vi "Vision Processing.vi"(8 "error in (no error)":errorcluster, 11 "Image Size":T1=enum."320x240") -> ()   [LabVIEW 2017]
uses:
  Vision Support Code/Camera Types.ctl
  <vilib>/Rock Robotics/WPI/Camera/WPI_CameraImageSize.ctl
  <vilib>/Rock Robotics/WPI/Camera/WPI_CameraWhite Balance Values.ctl
  <vilib>/Rock Robotics/WPI/Camera/WPI_CameraExposure Values.ctl
  <vilib>/Rock Robotics/WPI/Camera/WPI_CameraFrameRate.ctl
  Robot Global Data.vi
  <vilib>/Rock Robotics/Network Tables/NT Write Number.vi
  <vilib>/vision/NI_Vision_Development_Module.lvlib
panel:
  in  "Image Size 2":T1=enum."320x240"
  in  "Min Component %":dbl=15.0
  out "loop ms":u32
  in  "Display Original":bool
  in  "Display Mask":bool
  out "Instructions:":string="Connect a USB or IP camera to your roboRIO. If using a ring light and retroreflective tape, use Camera Settings outside the loop create a dark image with bright and colorful stripes. If used wihtout a ring light, brighten the images so that stripes are visible.\n\nLED Color can encoded as HSL or related color modes. Calibrate to the same color as the strips being reflected to the camera. Unlike the desktop example, this LED color must be set by hand. You can also put the calibration on the dashboard and send the LED Color to the RT code using Network Tables.\n\nThe Display buttons affects whether images are displayed on the panel. It takes quite a bit of CPU  to compress and transmit the images for display.\n\nAdjust Score Cutoff to make the code more or less picky. If the color is not very unique, you may need to increase the number of particles considered. The diagram uses a Size Limit to ignore colored things that are too small. You may need to adjust it if you are targetting from far away.\n\nResults give you the distance to the target, the center and box in a normalized (-1 to 1) and pixel coordinates.\n\nBe sure to read about setting camera exposure and brightness to help simplify your image and acquire color saturated images.\n\nThere are lots of comments on the diagram to explain the code."
  in  "Color Mode":u16(ring)=2 items=["RGB", "HSL", "HSV", "HSI"]
  in  "Particles":dbl=5.0
  in  "Score Cutoff %":dbl=75.0
  in  "Camera Type":T2=enum."MS HD3000 square"
  out "Result":T3 {"Score" format="%#_3g"; "Pixels"."Rectangle"."Numeric 5" format="%#_3g"; "Pixels"."Rectangle"."Numeric 3" format="%#_3g"; "Pixels"."Rectangle"."Numeric 2" format="%#_3g"; "Pixels"."Rectangle"."Numeric" format="%#_3g"; "Normalized"."Rectangle"."Numeric 5" format="%#_2g"; "Normalized"."Rectangle"."Numeric 3" format="%#_2g"; "Normalized"."Rectangle"."Numeric 2" format="%#_2g"; "Normalized"."Rectangle"."Numeric" format="%#_2g"; "Normalized"."Center"."?" format="%#_3g"; "Normalized"."Center"."?" format="%#_3g"; "Distance (ft)" format="%#_3g"}
  out "Qualified Particles":i32
  in  "LED Color":T4={"Hue"={107.81818389892578, 139.81818389892578}, "Sat"={176.07142857142858, 255.0}, "Val"={40.53571428571429, 255.0}} {"Hue" scale=0.0..255.0 scale format="%#_3g"}
  out "Mask":T5(plugin-control)
  out "Original Image":T5(plugin-control)
  # "Good target, distance ft"
  # "Bad target"
  # "Score in %"
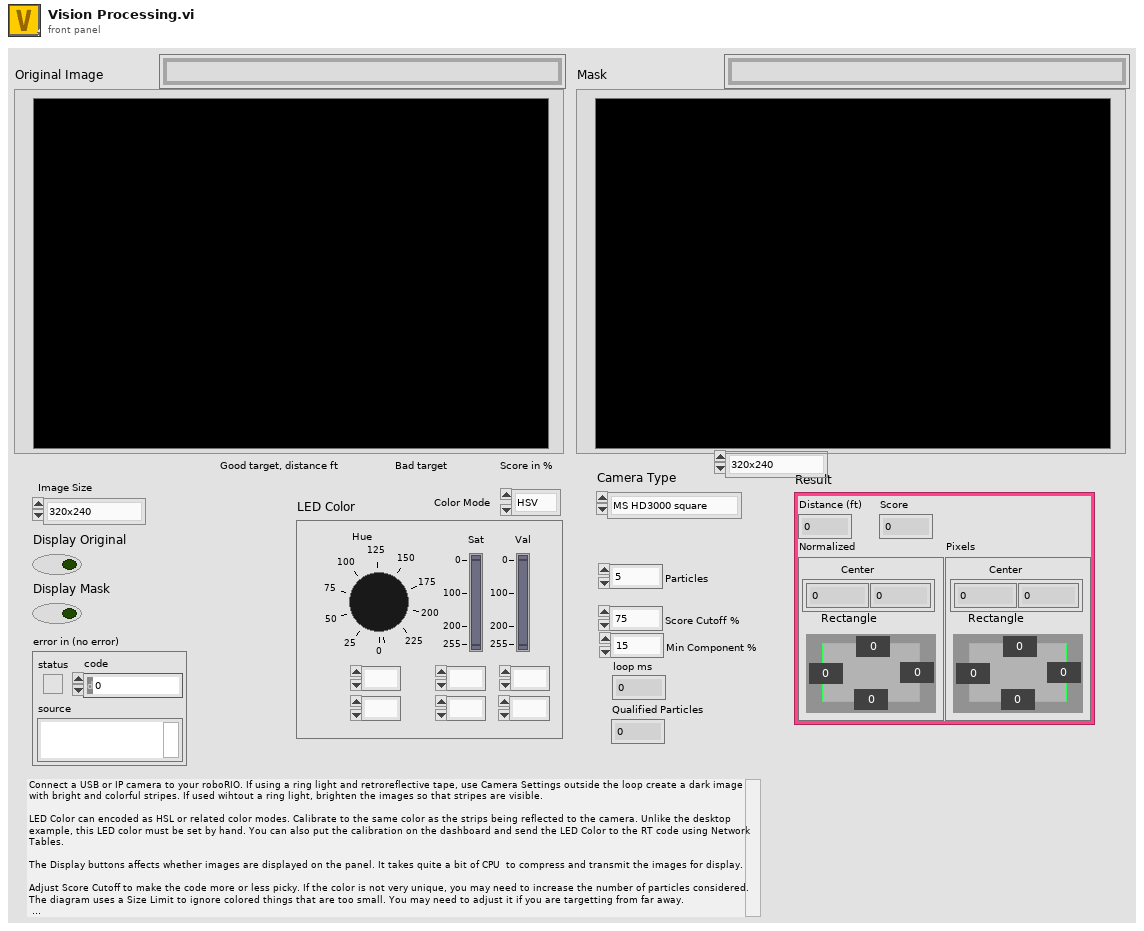
[diagram p1: front panel]
types:
  T1 = typedef "WPI_CameraImageSize.ctl" = enum16{"640x480", "320x240", "160x120", "Custom"}
  T2 = typedef "Camera Types.ctl" = enum16{"206", "1011", "1013", "MS HD3000 square", "MS HD3000 640x480"}
  T3 = cluster{"Distance (ft)":dbl, "Score":dbl, "Normalized":cluster{"Center":cluster{dbl, dbl}, "Rectangle":cluster{"Numeric":dbl, "Numeric 2":dbl, "Numeric 3":dbl, "Numeric 5":dbl}}, "Pixels":cluster{"Center":cluster{dbl, dbl}, "Rectangle":cluster{"Numeric":dbl, "Numeric 2":dbl, "Numeric 3":dbl, "Numeric 5":dbl}}}
  T4 = cluster{"Hue":cluster{dbl, dbl}, "Sat":cluster{dbl, dbl}, "Val":cluster{dbl, dbl}}
  T5 = typedef "IMAQ Image.ctl" = refnum<image>
  T6 = typedef "WPI_CameraFrameRate.ctl" = u32
  T7 = typedef "WPI_CameraExposure Values.ctl" = enum16{"Auto", "Flicker-free 50 Hz", "Flicker-free 60 Hz", "Hold current", "Custom"}
  T8 = typedef "WPI_CameraWhite Balance Values.ctl" = enum16{"Auto", "Fixed indoor", "Fixed outdoor 1", "Fixed outdoor 2", "Fixed fluorescent 1", "Fixed fluorescent 2", "Hold current", "Custom"}
  T9 = typedef "Particle Parameters" = i32
  T10 = typedef "Image Type" = u32
  T11 = typedef "WPI_CameraDevRef.ctl" = cluster{"Camera Address":string, "CameraStatus":errorcluster}
  T12 = cluster{"Score":dbl, "Rect":cluster{"Left":dbl, "Top":dbl, "Right":dbl, "Bottom":dbl}, "Full Scores":cluster{"Aspect Ratio":dbl, "Top Position":dbl, "Bottom Position":dbl, "Left Gap":dbl, "Width":dbl, "Height Ratio":dbl}}[]
  T13 = cluster{"Score":dbl, "Rect":cluster{"Left":dbl, "Top":dbl, "Right":dbl, "Bottom":dbl}, "Full Scores":cluster{"Aspect Ratio":dbl, "Top Position":dbl, "Bottom Position":dbl, "Left Gap":dbl, "Width":dbl, "Height Ratio":dbl}}
  T14 = cluster{"Left":dbl, "Top":dbl, "Right":dbl, "Bottom":dbl}
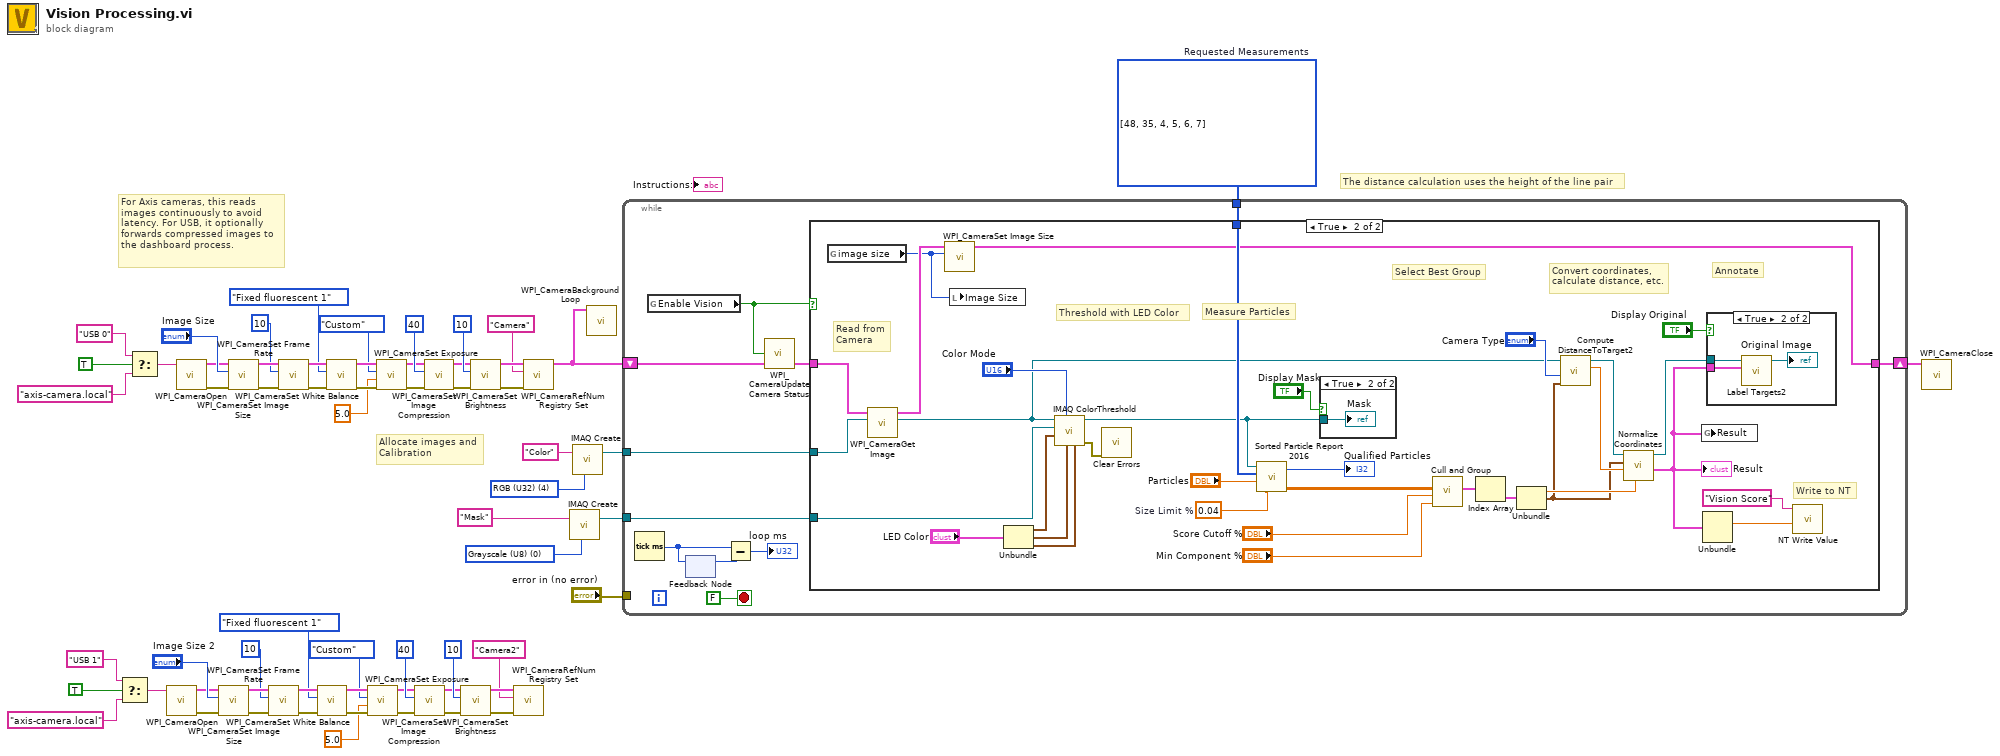
[diagram p0: block diagram]
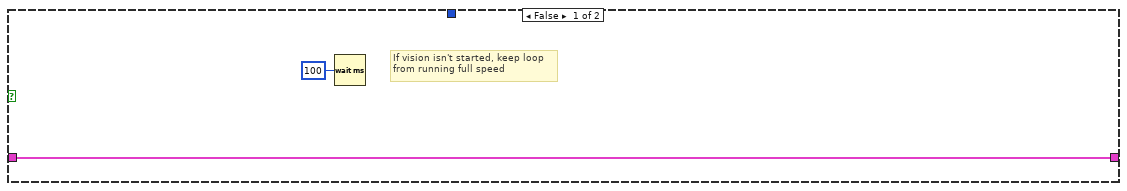
[diagram p2: hidden frame]
diagram:
  w57 = T9[] [48, 35, 4, 5, 6, 7] items=["Center of Mass X", "Center of Mass Y", "First Pixel X", "First Pixel Y", "Bounding Rect Left", "Bounding Rect Top", "Bounding Rect Right", "Bounding Rect Bottom", "Max Feret Diameter Start X", "Max Feret Diameter Start Y", "Max Feret Diameter End X", "Max Feret Diameter End Y", "Max Horiz. Segment Length Left", "Max Horiz. Segment Length Right", "Max Horiz. Segment Length Row", "-", "Bounding Rect Width", "Bounding Rect Height", "Bounding Rect Diagonal", "Perimeter", "Convex Hull Perimeter", "Holes' Perimeter", "Max Feret Diameter", "Equivalent Ellipse Major Axis", "Equivalent Ellipse Minor Axis", "Equivalent Ellipse Minor Axis (Feret)", "Equivalent Rect Long Side", "Equivalent Rect Short Side", "Equivalent Rect Diagonal", "Equivalent Rect Short Side (Feret)", "Average Horiz. Segment Length", "Average Vert. Segment Length", "Hydraulic Radius", "Waddel Disk Diameter", "-", "Area", "Holes' Area", "Particle & Holes' Area", "Convex Hull Area", "Image Area", "-", "Number of Holes", "Number of Horiz. Segments", "Number of Vert. Segments", "-", "Orientation", "Max Feret Diameter Orientation", "-", "% Area/Image Area", "% Area/(Particle & Holes' Area)", "Ratio of Equivalent Ellipse Axes", "Ratio of Equivalent Rect Sides", "-", "Elongation Factor", "Compactness Factor", "Heywood Circularity Factor", "Type Factor", "-", "Sum X", "Sum Y", "Sum XX", "Sum XY", "Sum YY", "Sum XXX", "Sum XXY", "Sum XYY", "Sum YYY", "-", "Moment of Inertia XX", "Moment of Inertia XY", "Moment of Inertia YY", "Moment of Inertia XXX", "Moment of Inertia XXY", "Moment of Inertia XYY", "Moment of Inertia YYY", "Norm. Moment of Inertia XX", "Norm. Moment of Inertia XY", "Norm. Moment of Inertia YY", "Norm. Moment of Inertia XXX", "Norm. Moment of Inertia XXY", "Norm. Moment of Inertia XYY", "Norm. Moment of Inertia YYY", "Hu Moment 1", "Hu Moment 2", "Hu Moment 3", "Hu Moment 4", "Hu Moment 5", "Hu Moment 6", "Hu Moment 7"]  # Requested Measurements
  w60 = T10 0 items=["Grayscale (U8)", "Grayscale (I16)", "Grayscale (SGL)", "Complex (CSG)", "RGB (U32)", "HSL (U32)", "RGB (U64)", "Grayscale (U16)"] ("Image Type")
  w61 = T10 4 items=["Grayscale (U8)", "Grayscale (I16)", "Grayscale (SGL)", "Complex (CSG)", "RGB (U32)", "HSL (U32)", "RGB (U64)", "Grayscale (U16)"] ("Image Type")
  # "For Axis cameras, this reads\nimages continuously to avoid\nlatency. For USB, it optionally\nforwards compressed images to\nthe dashboard process."
  # "The distance calculation uses the height of the line pair"
  # "Allocate images and\nCalibration"
  n1 = Select(t="USB 1" ("format string"), s=TRUE ("dot notation? (F)"), f="axis-camera.local" ("format string")) -> (s? t:f=w2:string)
  n2 = Select(t="USB 0" ("format string"), s=TRUE ("dot notation? (F)"), f="axis-camera.local" ("format string")) -> (s? t:f=w31:string)
  n3 = call <vilib>:"WPI_CameraOpen.vi"("Camera Address"=w2) -> ("error out"=w14:errorcluster, "CameraDevRef"=w15:T11)  [unwired: 2 in, 7 out]
  n4 = call <vilib>:"WPI_CameraOpen.vi"("Camera Address"=w31) -> ("error out"=w43:errorcluster, "CameraDevRef"=w44:T11)  [unwired: 2 in, 7 out]
  n5 = call <vilib>:"WPI_CameraSet Image Size.vi"("error in (no error)"=w14, "Image Size"="Image Size 2", "CameraDevRef"=w15) -> ("error out"=w13:errorcluster, "CameraDevRef Out"=w16:T11)  [unwired: 1 in, 6 out]
  n6 = call <vilib>:"WPI_CameraSet Image Size.vi"("error in (no error)"=w43, "Image Size"="Image Size", "CameraDevRef"=w44) -> ("error out"=w42:errorcluster, "CameraDevRef Out"=w45:T11)  [unwired: 1 in, 6 out]
  n7 = call <vilib>:"WPI_CameraSet Frame Rate.vi"("error in (no error)"=w13, "Frame Rate (fps)"=T6 10, "CameraDevRef"=w16) -> ("error out"=w12:errorcluster, "CameraDevRef Out"=w18:T11)  [unwired: 7 out]
  n8 = call <vilib>:"WPI_CameraSet Frame Rate.vi"("error in (no error)"=w42, "Frame Rate (fps)"=T6 10, "CameraDevRef"=w45) -> ("error out"=w41:errorcluster, "CameraDevRef Out"=w47:T11)  [unwired: 7 out]
  n9 = call <vilib>:"WPI_CameraSet White Balance.vi"("error in (no error)"=w12, "White Balance"=WPI_CameraWhite_Balance_Values."Fixed fluorescent 1", "CameraDevRef"=w18) -> ("error out"=w11:errorcluster, "CameraDevRef Out"=w17:T11)  [unwired: 1 in, 6 out]
  n10 = call <vilib>:"WPI_CameraSet White Balance.vi"("error in (no error)"=w41, "White Balance"=WPI_CameraWhite_Balance_Values."Fixed fluorescent 1", "CameraDevRef"=w47) -> ("error out"=w40:errorcluster, "CameraDevRef Out"=w46:T11)  [unwired: 1 in, 6 out]
  n11 = call <vilib>:"WPI_CameraSet Exposure.vi"("error in (no error)"=w11, "Exposure (%)"=5.0, "Exposure"=WPI_CameraExposure_Values."Custom", "CameraDevRef"=w17) -> ("error out"=w10:errorcluster, "CameraDevRef Out"=w20:T11)  [unwired: 6 out]
  n12 = call <vilib>:"WPI_CameraSet Exposure.vi"("error in (no error)"=w40, "Exposure (%)"=5.0, "Exposure"=WPI_CameraExposure_Values."Custom", "CameraDevRef"=w46) -> ("error out"=w39:errorcluster, "CameraDevRef Out"=w49:T11)  [unwired: 6 out]
  n13 = call <vilib>:"WPI_CameraSet Image Compression.vi"("error in (no error)"=w10, "Compression"=40, "CameraDevRef"=w20) -> ("error out"=w9:errorcluster, "CameraDevRef Out"=w19:T11)  [unwired: 7 out]
  n14 = call <vilib>:"WPI_CameraSet Image Compression.vi"("error in (no error)"=w39, "Compression"=40, "CameraDevRef"=w49) -> ("error out"=w38:errorcluster, "CameraDevRef Out"=w48:T11)  [unwired: 7 out]
  n15 = call <vilib>:"WPI_CameraSet Brightness.vi"("error in (no error)"=w9, "Brightness"=10, "CameraDevRef"=w19) -> ("error out"=w8:errorcluster, "CameraDevRef Out"=w26:T11)  [unwired: 1 in, 6 out]
  n16 = call <vilib>:"WPI_CameraSet Brightness.vi"("error in (no error)"=w38, "Brightness"=10, "CameraDevRef"=w48) -> ("error out"=w37:errorcluster, "CameraDevRef Out"=w55:T11)  [unwired: 1 in, 6 out]
  n17 = call <vilib>:"WPI_CameraRefNum Registry Set.vi"("error in (no error)"=w8, "refnum name"="Camera2", "CameraDevRef"=w26) -> ()  [unwired: 1 in, 8 out]
  n18 = call <vilib>:"WPI_CameraRefNum Registry Set.vi"("error in (no error)"=w37, "refnum name"="Camera", "CameraDevRef"=w55) -> ("CameraDevRef"=w30:T11)  [unwired: 1 in, 7 out]
  n19 = call "IMAQ Create"("Image Name"="Mask", "Image Type"=w60) -> ("New Image"=w58:T5)  [unwired: 2 in, 2 out]
  n20 = call "IMAQ Create"("Image Name"="Color", "Image Type"=w61) -> ("New Image"=w56:T5)  [unwired: 2 in, 2 out]
  n21 = call <vilib>:"WPI_CameraBackground Loop.vi"("CameraDevRef"=w30) -> ()  [unwired: 11 in]
  n22 = while {
    tunnel: w56 -> [w70]
    tunnel: w58 -> [w72]
    tunnel: w57 -> [w71]
    shift-right: [w69] -> w29
    shift-left: w30 -> [w68]
    tunnel: "error in (no error)" -> [_]
    stop <- FALSE stop-if-true
    n23 = Tick Count (ms)() -> (millisecond timer value=w64:u32)
    n24 = global read "Robot Global Data.vi" "Enable Vision"() -> (w66:bool)
    n25 = feedback-in #1(w64) -> ()
    n26 = feedback #1() -> (w65:u32)  [unwired: 1 in]
    n27 = Subtract(x=w64, y=w65) -> (x-y=→"loop ms":u32)
    n28 = call <vilib>:"WPI_CameraUpdate Camera Status.vi"("CameraDevRef In"=w68, "Enable Vision"=w66) -> ("CameraDevRef Out"=w67:T11)  [unwired: 3 in]
    n29 = case shown="True" w66 {
      tunnel: w72 -> [_ w109]
      tunnel: w71 -> [_ w105]
      tunnel: w67 -> [w75 w91]
      tunnel: w70 -> [_ w90]
      tunnel: [w75 w85] -> w69
      frame False {
        # "If vision isn't started, keep loop\nfrom running full speed"
        n30 = Wait (ms)(milliseconds to wait=u32 100) -> ()  [unwired: 1 out]
      }
      frame True {
        w103 = 0.04  # Size Limit %
        # "Write to NT"
        # "Read from\nCamera"
        # "Measure Particles"
        # "Convert coordinates,\ncalculate distance, etc."
        # "Annotate"
        # "Select Best Group"
        # "Threshold with LED Color"
        n31 = global read "Robot Global Data.vi" "image size"() -> (w84:T1)
        n32 = call <vilib>:"WPI_CameraGet Image.vi"("Image"=w90, "CameraDevRef"=w91) -> ("Image Out"=w89:T5, "CameraDevRef Out"=w86:T11)  [unwired: 7 in, 1 out]
        n33 = call <vilib>:"WPI_CameraSet Image Size.vi"("Image Size"=w84, "CameraDevRef"=w86) -> ("CameraDevRef Out"=w85:T11)  [unwired: 2 in, 7 out]
        n34 = local write "Image Size"(w84) -> ()
        n35 = Unbundle("LED Color") -> ("Hue"=w108:cluster{dbl, dbl}, "Sat"=w107:cluster{dbl, dbl}, "Val"=w106:cluster{dbl, dbl})
        n36 = call "IMAQ ColorThreshold"("Blue or Luma or Val or Inten Range"=w106, "Green or Sat Range"=w107, "Color Mode"="Color Mode", "Red or Hue Range"=w108, "Image Dst"=w109, "Image Src"=w89) -> ("error out"=w102:errorcluster, "Image Dst Out"=w98:T5)  [unwired: 4 in]
        n37 = call <vilib>:"Clear Errors.vi"("error in (no error)"=w102) -> ()  [unwired: 5 in, 2 out]
        n38 = call "Sorted Particle Report 2016.vi"("Min Area Size %"=w103, "Particle Count Limit"="Particles", "Pixel Measurements"=w105, "Image in"=w98) -> ("Sorted Data"=w100:dbl[][], "Particles"=→"Qualified Particles":i32)
        n39 = case shown="True" "Display Mask" {
          tunnel: w98 -> [_ w113]
          frame False {
          }
          frame True {
            "Mask" <- w113
          }
        }
        n40 = call "Cull and Group.vi"("Min Compnt %"="Min Component %", "Score Cutoff %"="Score Cutoff %", "Sorted Data"=w100) -> ("Best Targets above cutoff"=w80:T12)  [unwired: 8 in]
        n41 = Index Array(array=w80) -> (element=w79:T13)  [unwired: 1 in]
        n42 = Unbundle(w79) -> ("Score"=w78:dbl, "Rect"=w77:T14)  [unwired: 1 out]
        n43 = call "Compute DistanceToTarget2.vi"("Rect"=w77, "Camera Type"="Camera Type", "Image Src"=w89) -> ("Distance (ft)"=w96:dbl, "Image Dst Out"=w95:T5)  [unwired: 7 in]
        n44 = call "Normalize Coordinates.vi"("Score"=w78, "Distance"=w96, "Bounding box"=w77, "Image in"=w95) -> ("Results"=w83:T3, "Image out"=w94:T5)  [unwired: 6 in]
        "Result" <- w83
        n45 = global write "Robot Global Data.vi" "Result"(w83) -> ()
        n46 = Unbundle(w83) -> ("Score"=w82:dbl)  [unwired: 3 out]
        n47 = case shown="True" "Display Original" {
          tunnel: w94 -> [_ w111]
          tunnel: w83 -> [_ w110]
          frame False {
          }
          frame True {
            n48 = call "Label Targets2.vi"("Results"=w110, "Image in"=w111) -> ("Image out"=→"Original Image":T5)  [unwired: 9 in]
          }
        }
        n49 = call-poly <vilib>:"NT Write Value.vi"("Numeric"=w82, "Name"="Vision Score") -> ()  [unwired: 9 in, 1 out]
      }
    }
  }
  n50 = call <vilib>:"WPI_CameraClose.vi"("CameraDevRef"=w29) -> ()  [unwired: 1 in, 10 out]
